vi "Save Recall Setup.vi"(8 "error in (no error)":errorcluster, 9 "setup number (0)":i32 min=0 max=9 step=1, 10 "mode (0:Save)":u16(ring) items=["Save", "Recall"], 11 "VISA resource name":refnum<visa-resource-name>) -> (0 "error out":errorcluster, 3 "VISA resource name out":refnum<visa-resource-name>)   [LabVIEW 2016, in "Agilent 4263X.lvlib"]
doc: "This VI saves or recalls instrument setups."
uses:
  <instrlib>/Agilent 4263X/Agilent 4263X.lvlib
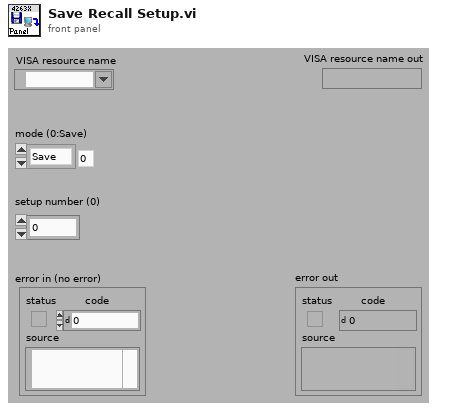
[diagram p1: front panel]
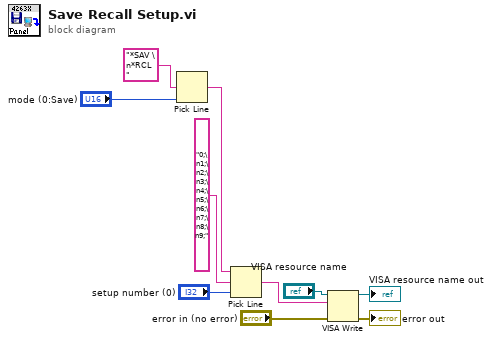
[diagram p0: block diagram]
diagram:
  n1 = Pick Line(multi-line string="*SAV \n*RCL ", line index="mode (0:Save)") -> (output string=w5:string)  [unwired: 1 in]
  n2 = Pick Line(string ("")=w5, multi-line string="0;\n1;\n2;\n3;\n4;\n5;\n6;\n7;\n8;\n9;", line index="setup number (0)") -> (output string=w1:string)
  n3 = VISA Write(VISA resource name="VISA resource name", write buffer=w1, error in (no error)="error in (no error)") -> (VISA resource name out=→"VISA resource name out":refnum<visa-resource-name>, error out=→"error out":errorcluster)  [unwired: 1 out]
